vi "open_h264.vi"(8 "error in (no error)":errorcluster, 9 "height":i32, 10 "width":i32, 11 "filename":path) -> (0 "error out":errorcluster, 3 "h264_file_handle":u64)   [LabVIEW 2011, in "librir.lvlib"]
uses:
  librir.lvlib
  libs/video_io.dll
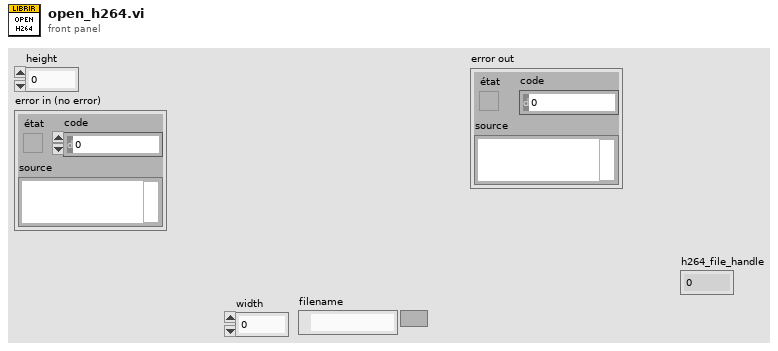
[diagram p1: front panel]
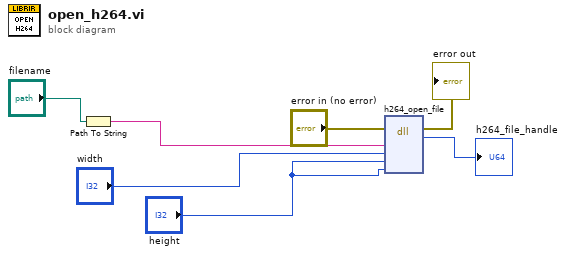
[diagram p0: block diagram]
diagram:
  n1 = Path To String(path="filename") -> (string=w4:string)
  n2 = dll-call lib="G:/librir/src/labview/libs/video_io.dll" fn="h264_open_file"(error in="error in (no error)", "filename"=w4, "width"="width", "height"="height", "lossy_height"="height") -> (error out=→"error out":errorcluster, "ir_file_handler"=→"h264_file_handle":u64)  [unwired: 6 in, 1 out]
